vi "温度曲线写入.vi"(8 "error in (no error)":errorcluster caption="错误输入（无错误）", 10 "data":T1={"时间"=timestamp(0 s since 1904-01-01), "测量模式"="水样测试", "数据类型"="N", "检测值"=0.0, "单位"="mg/L", "数据标识"="N", "X"=0.0, "量程标识"="", "SN"="", "标样参考值"=0.0, "跨度值"=0.0, "F0"=0.0, "F1"=0.0, "F2"=0.0, "F3"=0.0, "F4"=0.0, "F5"=0.0, "F6"=0.0, "F7"=0.0, "X1"=0.0, "因子编码"="", "温度"=0.0, "湿度"=0.0, "测量量程"=0.0, "测量检出限"=0.0, "测量精度"=0.0, "测量间隔"=0.0, "消解温度"=0.0, "消解时长"=0.0, "三项式系数"=0.0, "二次多项式系数"=0.0, "曲线斜率"=0.0, "曲线截距"=0.0, "线性相关系数"=0.0, "空白校准时间"=timestamp(0 s since 1904-01-01), "标样校准时间"=timestamp(0 s since 1904-01-01), "测量信号值"=0.0, "稀释倍数"=0.0, "空白标定系数"=0.0, "量程系数"=0.0, "LastTime"=timestamp(0 s since 1904-01-01)}, 11 "table":string="总氮") -> (0 "错误输出":errorcluster)   [LabVIEW 2016, in "斯坦道CODcr.lvlib"]
uses:
  <vilib>/Utility/VariantDataType/VariantType.lvlib
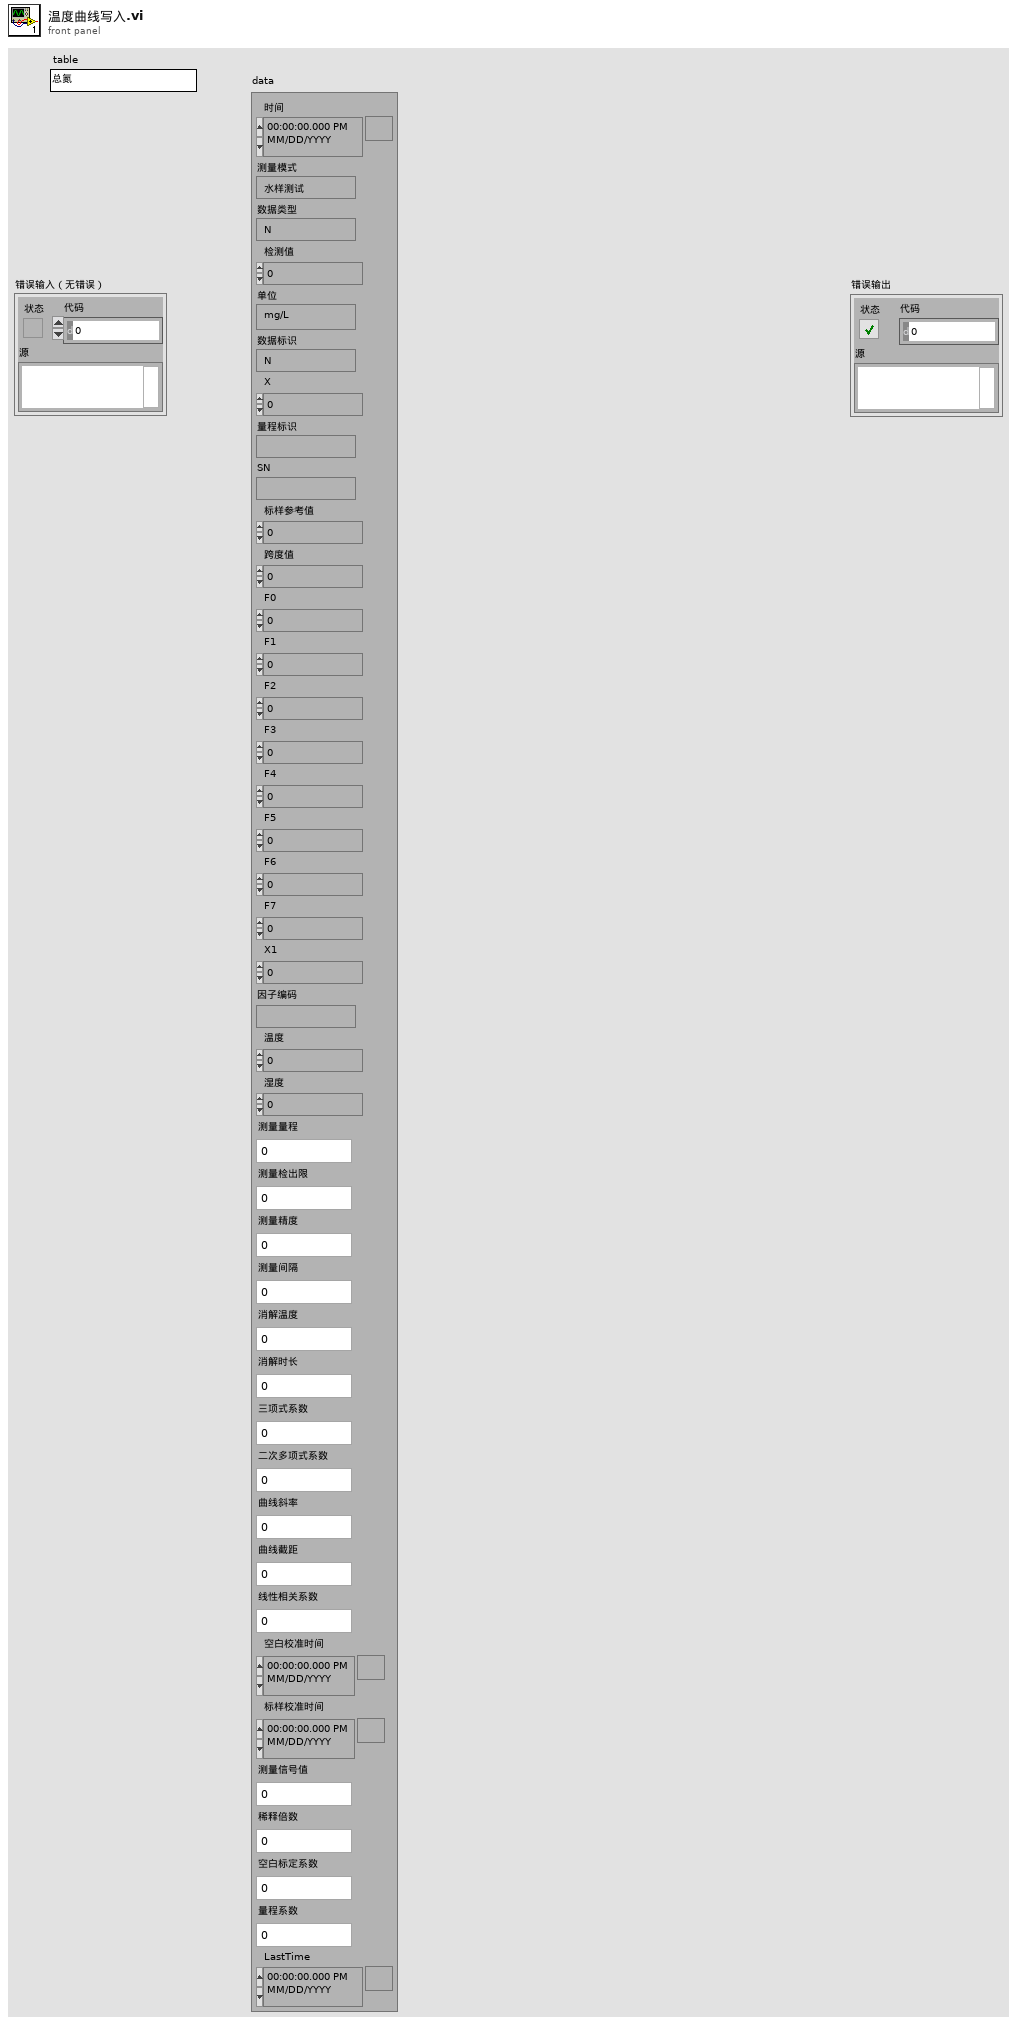
[diagram p1: front panel]
types:
  T1 = typedef "营养盐字段定义.ctl" = cluster{"时间":timestamp, "测量模式":string, "数据类型":string, "检测值":sgl, "单位":string, "数据标识":string, "X":sgl, "量程标识":string, "SN":string, "标样参考值":sgl, "跨度值":sgl, "F0":sgl, "F1":sgl, "F2":sgl, "F3":sgl, "F4":sgl, "F5":sgl, "F6":sgl, "F7":sgl, "X1":sgl, "因子编码":string, "温度":sgl, "湿度":sgl, "测量量程":sgl, "测量检出限":sgl, "测量精度":sgl, "测量间隔":sgl, "消解温度":sgl, "消解时长":sgl, "三项式系数":sgl, "二次多项式系数":sgl, "曲线斜率":sgl, "曲线截距":sgl, "线性相关系数":sgl, "空白校准时间":timestamp, "标样校准时间":timestamp, "测量信号值":sgl, "稀释倍数":sgl, "空白标定系数":sgl, "量程系数":sgl, "LastTime":timestamp}
  T2 = enum16{"open", "open or create", "create or replace", "create", "open (read-only)"}
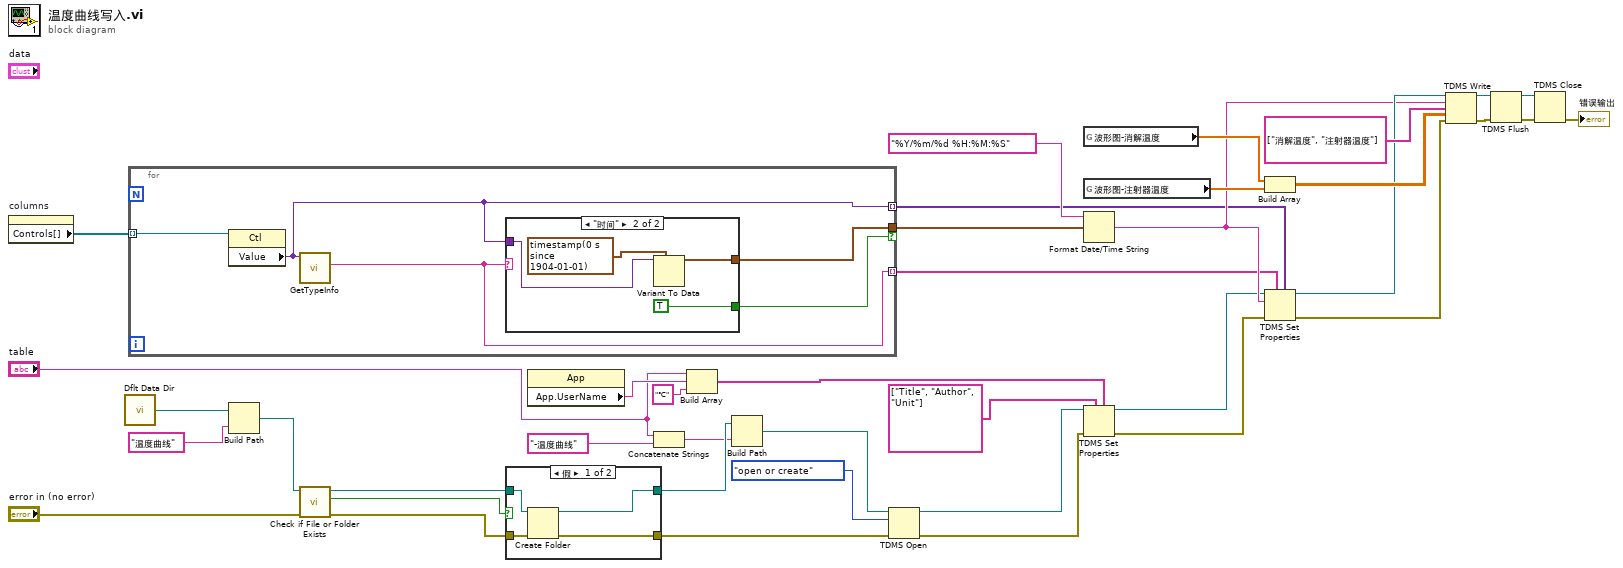
[diagram p0: block diagram]
diagram:
  n1 = property on="columns" class="Clust (严格)"() -> ("Controls[]"=w1:refnum<vi>[])  [unwired: 2 in, 2 out]
  n2 = call <vilib>:"Dflt Data Dir.vi"() -> ("App:Default Data Directory"=w29:path)
  n3 = for {
    tunnel: [w40] -> w4 mode=indexing
    tunnel: [w44] -> w5 mode=indexing
    tunnel: [w43] -> w2 if=w42
    tunnel: w1 -> [w41] mode=indexing
    n4 = property class="Ctl"(reference=w41) -> ("Value"=w40:variant)  [unwired: 1 in, 2 out]
    n5 = call <vilib>:"GetTypeInfo.vi"("Variant"=w40) -> ("Name"=w44:string)  [unwired: 6 in, 4 out]
    n6 = case shown="\"时间\"" w44 {
      tunnel: w40 -> [_ w48]
      tunnel: [_ w46] -> w43
      tunnel: [_ TRUE] -> w42
      frame "假", Default {
      }
      frame "时间" {
        n7 = Variant To Data(type=timestamp(0 s since 1904-01-01) ("时间标识"), Variant=w48) -> (data=w46:timestamp)  [unwired: 1 in, 1 out]
      }
    }
  }
  n8 = Build Path(base path=w29, name or relative path="温度曲线" ("名称或相对路径")) -> (appended path=w27:path)
  n9 = call <vilib>:"Check if File or Folder Exists.vi"("error in (no error)"="error in (no error)", "path"=w27) -> ("error out"=w24:errorcluster, "file or folder exists?"=w26:bool, "dup path"=w25:path)  [unwired: 7 in]
  n10 = case shown="假" w26 {
    tunnel: w25 -> [w52 w53]
    tunnel: [w51 w53] -> w23
    tunnel: w24 -> [w50 w54]
    tunnel: [w49 w54] -> w13
    frame False {
      n11 = Create Folder(path (use dialog)=w52, error in=w50) -> (created path=w51:path, error out=w49:errorcluster)  [unwired: 1 in, 1 out]
    }
    frame True {
    }
  }
  n12 = property class="App"() -> ("App.UserName"=w38:string)  [unwired: 2 in, 2 out]
  n13 = Concatenate Strings("table", "-温度曲线" ("字符串")) -> (w21:string)
  n14 = Build Array("table", w38, "℃" ("元素")) -> (w36:string[])
  n15 = Build Path(base path=w23, name or relative path=w21) -> (appended path=w20:path)
  n16 = TDMS Open(8:w13, 10:T2."open or create" ("操作(0:open)"), 11:w20) -> (0:w39:errorcluster, 3:w3:refnum<k34>)  [unwired: 4 in]
  n17 = global read "VAR总磷总氮全局变量.vi" "波形图-消解温度"() -> (w31:dbl[])
  n18 = global read "VAR总磷总氮全局变量.vi" "波形图-注射器温度"() -> (w30:dbl[])
  n19 = Format Date/Time String(time format string (%c)="%Y/%m/%d %H:%M:%S" ("时间格式字符串(%c)"), seconds (now)=w2) -> (date/time string=w15:string)  [unwired: 1 in]
  n20 = TDMS Set Properties(5:w36, 7:string[] ["Title", "Author", "Unit"] ("property names"), 8:w39, 11:w3) -> (0:w18:errorcluster, 3:w6:refnum<k34>)  [unwired: 2 in, 2 out]
  n21 = Build Array(w31, w30) -> (w34:dbl[][])
  n22 = TDMS Set Properties(5:w4, 7:w5, 8:w18, 10:w15, 11:w6) -> (0:w17:errorcluster, 3:w16:refnum<k34>)  [unwired: 1 in, 2 out]
  n23 = TDMS Write(0:w16, 5:w15, 7:string[] ["消解温度", "注射器温度"] ("通道名输入（无标题）"), 9:w34, 11:w17) -> (4:w10:refnum<k34>, 15:w9:errorcluster)  [unwired: 1 in, 2 out]
  n24 = TDMS Flush(4:w9, 7:w10) -> (0:w8:errorcluster, 3:w7:refnum<k34>)
  n25 = TDMS Close(8:w8, 11:w7) -> (0:→"错误输出":errorcluster)  [unwired: 1 out]
